vi "Configure Math Function (FFT Detector).vi"(4 "Math Function Index (1: Math Function 1)":i32(ring)=1 items=["Math Function 1"=1, "Math Function 2"=2, "Math Function 3"=3, "Math Function 4"=4], 8 "error in (no error)":errorcluster, 9 "Maximum Points (640)":i32=640, 10 "Detector Type (0: Off)":i32(ring) items=["Off", "Sample", "Positive (+Peak)", "Negative (-Peak)", "Normal", "Average"], 11 "VISA resource name":refnum<visa-resource-name>) -> (0 "error out":errorcluster, 3 "VISA resource name out":refnum<visa-resource-name>)   [LabVIEW 2015, in "Agilent 2000 3000 X-Series.lvlib"]
doc: "Configures the math function FFT detector.\n\n<b>Note:</b>\n - This VI is applicable for 3000T, 4000, 6000 Series."
uses:
  Agilent 2000 3000 X-Series.lvlib
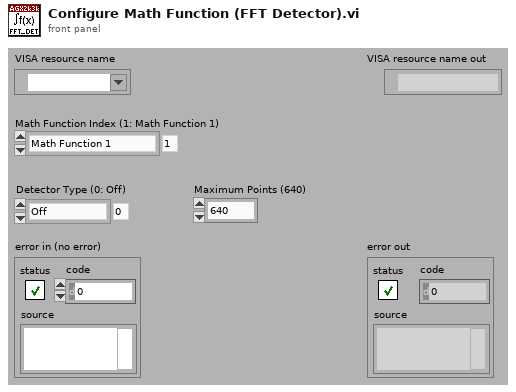
[diagram p1: front panel]
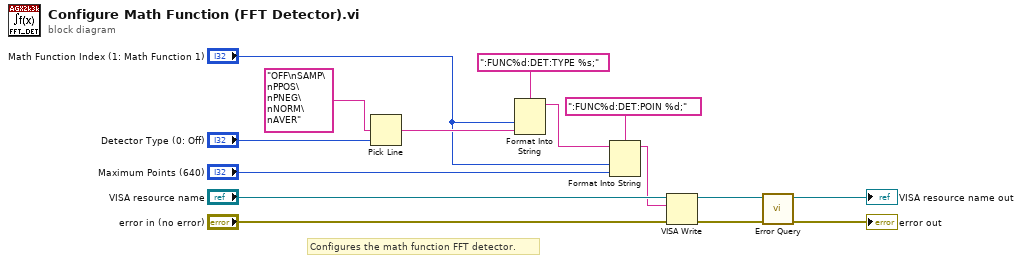
[diagram p0: block diagram]
diagram:
  # "Configures the math function FFT detector."
  n1 = Pick Line(multi-line string="OFF\nSAMP\nPPOS\nPNEG\nNORM\nAVER", line index="Detector Type (0: Off)") -> (output string=w5:string)  [unwired: 1 in]
  n2 = Format Into String(format string=":FUNC%d:DET:TYPE %s;", "Math Function Index (1: Math Function 1)", w5) -> (resulting string=w2:string)  [unwired: 2 in, 1 out]
  n3 = Format Into String(format string=":FUNC%d:DET:POIN %d;", initial string=w2, "Math Function Index (1: Math Function 1)", "Maximum Points (640)") -> (resulting string=w1:string)  [unwired: 1 in, 1 out]
  n4 = VISA Write(VISA resource name="VISA resource name", write buffer=w1, error in (no error)="error in (no error)") -> (VISA resource name out=w9:refnum<visa-resource-name>, error out=w8:errorcluster)  [unwired: 1 out]
  n5 = call "Error Query.vi"("error in (no error)"=w8, "VISA resource name"=w9) -> ("error out"=→"error out":errorcluster, "VISA resource name out"=→"VISA resource name out":refnum<visa-resource-name>)  [unwired: 6 in, 2 out]
